vi "GE 5565PIORC.PIO.Read In-Place (1D Bool).vi"(5 "count (-1: all)":i32=-1, 7 "byte order (big-endian)":T1(ring), 8 "error in (no error)":errorcluster, 9 "data in":bool[](array[boolean]), 10 "offset":u32, 11 "GE 5565PIORC in":refnum<class "GE 5565PIORC.lvclass">) -> (0 "error out":errorcluster, 1 "data out":bool[](array[boolean]), 3 "GE 5565PIORC out":refnum<class "GE 5565PIORC.lvclass">)   [LabVIEW 2016, in "GE 5565PIORC.lvclass"]
doc: "Reads <B>count</B> elements of <B>data</B> from the specified <B>offset</B>. The number of elements transferred will be either <B>count</B> or the number of elements in <B>data</B>, whichever is smaller."
uses:
  GE 5565PIORC.lvclass
  <vilib>/Instr/_visa.llb/VISA Register Access Address Space.ctl
  GE 5565PIORC.lvclass/GE 5565PIORC.ctl
  GE 5565PIORC.VISA.Move In-Place.String (U8).vi
  GE 5565PIORC.VISA.Return Handler.vi
  <vilib>/Utility/error.llb/Error Cluster From Error Code.vi
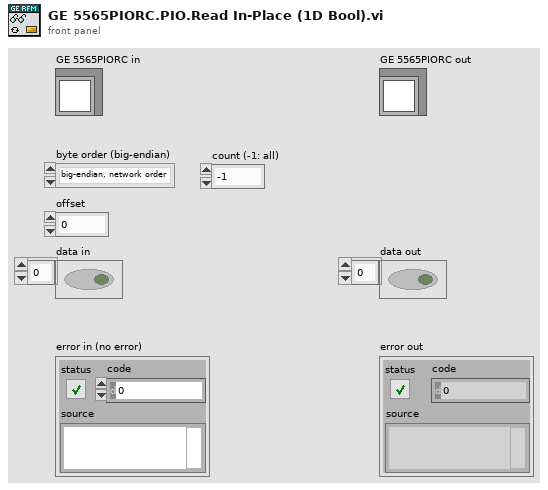
[diagram p1: front panel]
types:
  T1 = enum16{"big-endian, network order", "native, host order", "little-endian"}
  T2 = typedef "VISA Register Access Address Space.ctl" = u16
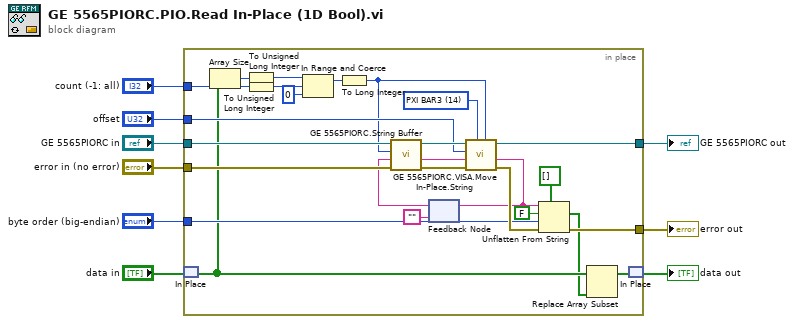
[diagram p0: block diagram]
diagram:
  n1 = in-place {
    in-place-border: "error in (no error)" -> [w25]
    in-place-border: [w35] -> w8
    in-place-border: "GE 5565PIORC in" -> [w26]
    in-place-border: "offset" -> [w16]
    in-place-border: "byte order (big-endian)" -> [w20]
    in-place-border: [w29] -> w4
    in-place-border: "count (-1: all)" -> [w18]
    w30 = T2 14 items=["VXI/VME A16"=1, "VXI/VME A24"=2, "VXI/VME A32"=3, "VXI/VME A64"=4, "PXI Memory Allocations"=9, "PXI Configuration"=10, "PXI BAR0"=11, "PXI BAR1"=12, "PXI BAR2"=13, "PXI BAR3"=14, "PXI BAR4"=15, "PXI BAR5"=16] ("address space")
    n2 = in-place-match #1("data in") -> (w15:bool[])
    n3 = Array Size(array=w15) -> (size(s)=w32:i32)
    n4 = To Unsigned Long Integer(number=w32) -> (unsigned 32bit integer=w14:u32)
    n5 = To Unsigned Long Integer(number=w18) -> (unsigned 32bit integer=w13:u32)
    n6 = In Range and Coerce(upper limit=w14, x=w13, lower limit=u32 0) -> (coerced(x)=w17:u32)  [unwired: 1 out]
    n7 = To Long Integer(number=w17) -> (32bit integer=w11:i32)
    n8 = feedback #2("" ("data out")) -> (w21:string)
    n9 = call "GE 5565PIORC.String Buffer.vi"("error in (no error)"=w25, "string buffer in"=w21, "minimum size"=w11, "GE 5565PIORC in"=w26) -> ("error out"=w24:errorcluster, "string buffer out"=w23:string, "GE 5565PIORC out"=w27:refnum<class "GE 5565PIORC.lvclass">)  [unwired: 5 in]
    n10 = call-poly "GE 5565PIORC.VISA.Move In-Place.String.vi"("count (-1: all)"=w11, "address space"=w30, "error in (no error)"=w24, "data in"=w23, "offset"=w16, "GE 5565PIORC in"=w27) -> ("error out"=w28:errorcluster, "data out"=w22:string, "GE 5565PIORC out"=w29:refnum<class "GE 5565PIORC.lvclass">)  [unwired: 3 in]
    n11 = feedback-in #2(w22) -> ()
    n12 = Unflatten From String(type=bool[] [], binary string=w22, data includes array or string size? (T)=FALSE, byte order (0:big-endian, network order)=w20, error in (no error)=w28) -> (value=w12:bool[], error out=w35:errorcluster)  [unwired: 1 out]
    n13 = Replace Array Subset(array=w15, new element=w12) -> (w31:bool[])  [unwired: 1 in]
    n14 = in-place-match #1(w31) -> (→"data out":bool[])
  }
  "GE 5565PIORC out" <- w4
  "error out" <- w8
